vi "Pressure Test Manual.vi"() -> ()   [LabVIEW 2015]
uses:
  <vilib>/DAQmx/write.llb/DAQmx Write (Analog DBL 1Chan 1Samp).vi
  <vilib>/DAQmx/read.llb/DAQmx Read (Analog DBL 1Chan 1Samp).vi
  <vilib>/DAQmx/miscellaneous.llb/DAQmx Fill In Error Info.vi
panel:
  out "mA":dbl
  out "error out":errorcluster
  out "NI-DAQ Pressure":dbl
  in  "Desired PSI":dbl
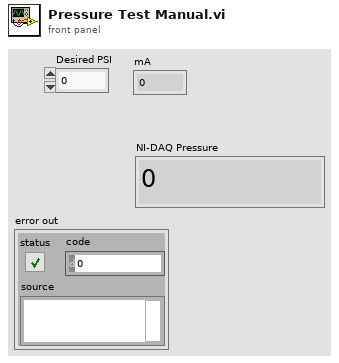
[diagram p1: front panel]
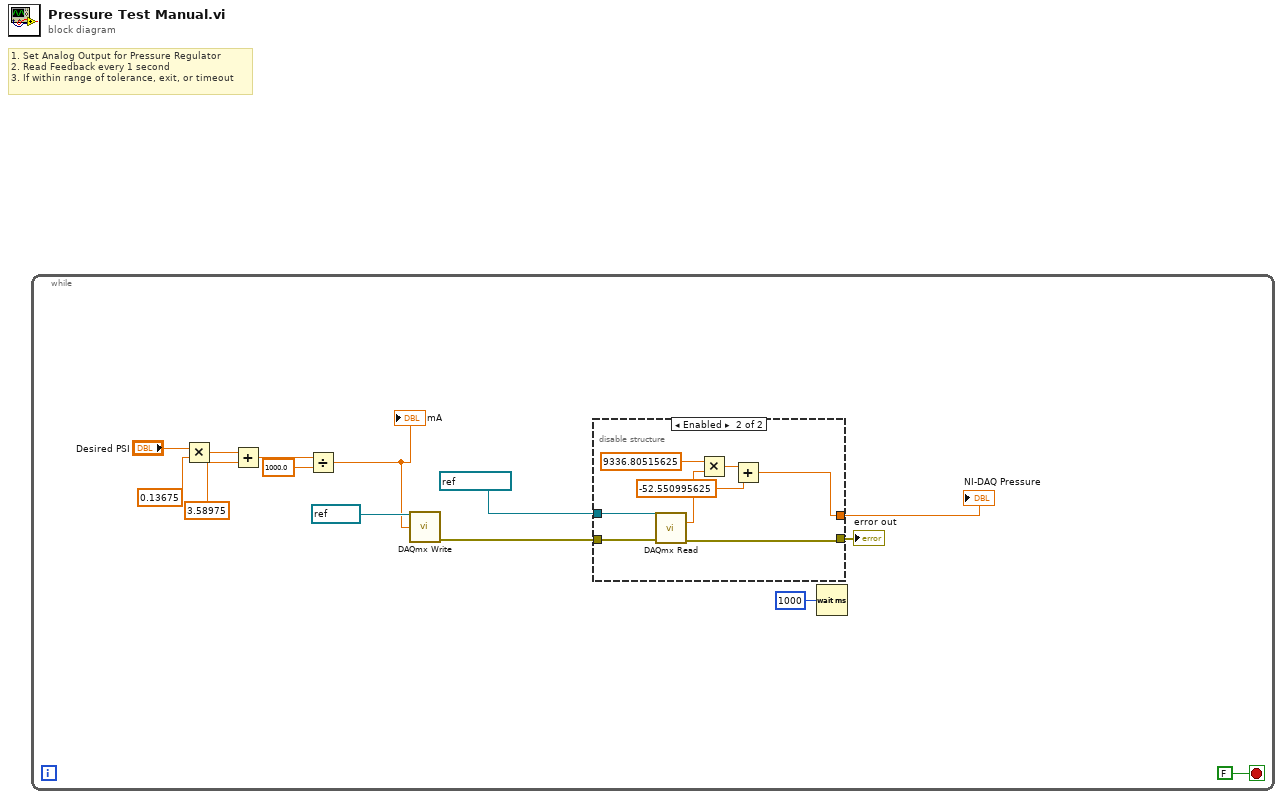
[diagram p0: block diagram]
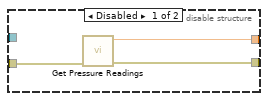
[diagram p2: hidden frame]
diagram:
  # "1. Set Analog Output for Pressure Regulator\n2. Read Feedback every 1 second\n3. If within range of tolerance, exit, or timeout"
  n1 = while {
    stop <- FALSE stop-if-true
    n2 = Multiply(x="Desired PSI", y=0.13675) -> (x*y=w13:dbl)
    n3 = Add(x=w13, y=3.58975) -> (x+y=w10:dbl)
    n4 = Divide(x=w10, y=1000.0) -> (x/y=w8:dbl)
    "mA" <- w8
    n5 = call-poly <vilib>:"DAQmx Write.vi"("task/channels in"=refnum<k21> "REG", "data"=w8) -> ("error out"=w6:errorcluster)  [unwired: 11 in, 2 out]
    n6 = disable-structure shown="Enabled" {
      disable-tunnel: w6 -> [w17 w25]
      disable-tunnel: [w16 w24] -> w1
      disable-tunnel: [w15 w18] -> w3
      disable-tunnel: refnum<k21> "Pressure" -> [_ w23]
      frame Disabled {
        n7 = call "Get Pressure Readings.vi"("error in (no error)"=w17) -> ("error out"=w16:errorcluster, "NI-DAQ Pressure"=w15:dbl)  [unwired: 7 in, 2 out]
      }
      frame Enabled {
        n8 = call-poly <vilib>:"DAQmx Read.vi"("task/channels in"=w23, "error in"=w25) -> ("data"=w22:dbl, "error out"=w24:errorcluster)  [unwired: 11 in, 1 out]
        n9 = Multiply(x=9336.80515625, y=w22) -> (x*y=w20:dbl)
        n10 = Add(x=w20, y=-52.550995625) -> (x+y=w18:dbl)
      }
    }
    "NI-DAQ Pressure" <- w3
    "error out" <- w1
    n11 = Wait (ms)(milliseconds to wait=u32 1000) -> ()  [unwired: 1 out]
  }
